vi "Find Sparks with RF Start Signal.vi"(3 "error in (no error)":errorcluster, 4 "Min Spark Length":i32=5000, 5 "Waveform":dbl[](array[numeric])) -> (0 "error out":errorcluster, 2 "Spark Indicies":i32[](array[numeric]))   [LabVIEW 2012]
panel:
  out "Waveform Graph":dbl[](graph)
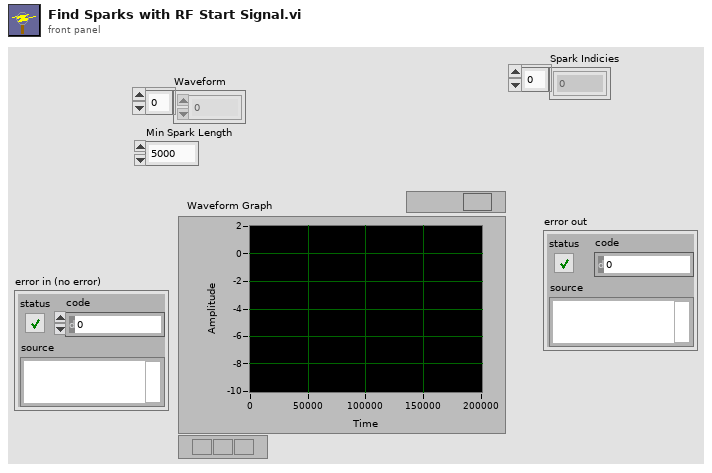
[diagram p1: front panel]
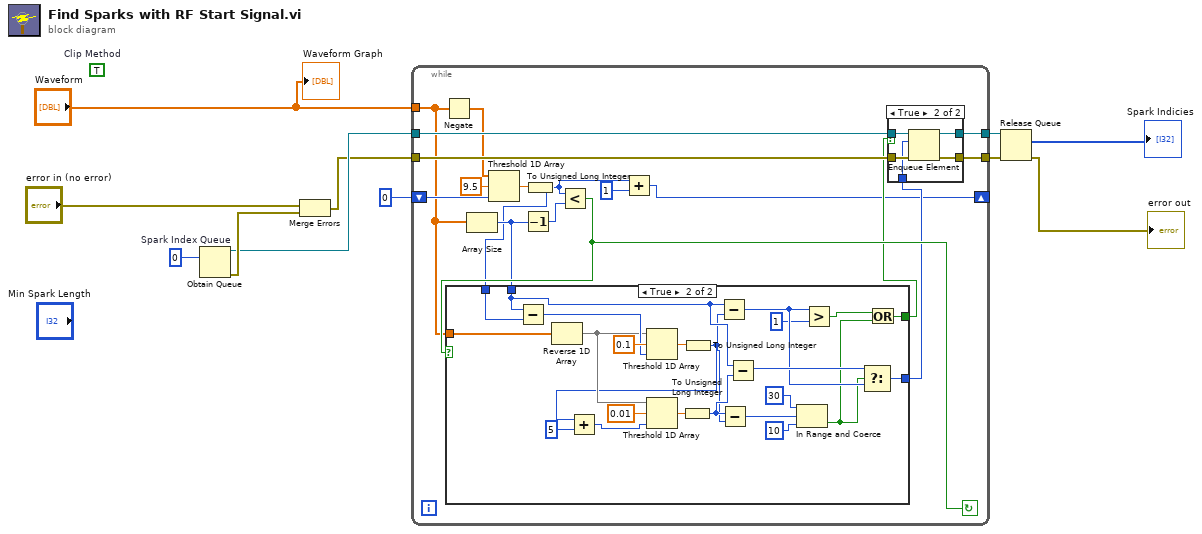
[diagram p0: block diagram]
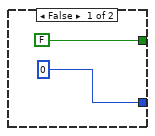
[diagram p3: hidden frame]
diagram:
  (unwired) TRUE  # Clip Method
  n1 = Obtain Queue "Spark Index Queue"(element data type=0 ("# Cluster Levels")) -> (queue out=w6:refnum<queue>, error out=w10:errorcluster)  [unwired: 4 in, 1 out]
  n2 = Merge Errors("error in (no error)", w10) -> (w5:errorcluster)
  n3 = while {
    tunnel: "Waveform" -> [w19]
    shift-right: [w12] -> _
    shift-left: 0 ("start index (0)") -> [w25]
    tunnel: w6 -> [w24]
    tunnel: w5 -> [w23]
    tunnel: [w22] -> w4
    tunnel: [w21] -> w3
    stop <- w20 continue-if-true
    n4 = Negate(x=w19) -> (-x=w15:dbl[])
    n5 = Array Size(array=w19) -> (size(s)=w18:i32)
    n6 = Threshold 1D Array(1:w25, 2:9.5 ("Voltage\nThreshold"), 3:w15) -> (0:w28:dbl)
    n7 = Decrement(x=w18) -> (x-1=w27:i32)
    n8 = To Unsigned Long Integer(number=w28) -> (unsigned 32bit integer=w14:u32)
    n9 = Less?(x=w14, y=w27) -> (x < y?=w20:bool)
    n10 = case shown="True" w20 {
      tunnel: w14 -> [_ w60]
      tunnel: w19 -> [_ w56]
      tunnel: w18 -> [_ w52]
      tunnel: [FALSE w43] -> w17
      tunnel: [u32 0 w46] -> w16
      frame False {
      }
      frame True {
        n11 = Subtract(x=w52, y=w60) -> (x-y=w57:u32)
        n12 = Reverse 1D Array(array=w56) -> (reversed array=w54:dbl[])
        n13 = Threshold 1D Array(1:w57, 2:0.1 ("threshold y"), 3:w54) -> (0:w58:dbl)
        n14 = To Unsigned Long Integer(number=w58) -> (unsigned 32bit integer=w39:u32)
        n15 = Add(x=w39, y=u32 5) -> (x+y=w40:u32)
        n16 = Threshold 1D Array(1:w40, 2:0.01 ("threshold y"), 3:w54) -> (0:w53:dbl)
        n17 = To Unsigned Long Integer(number=w53) -> (unsigned 32bit integer=w51:u32)
        n18 = Subtract(x=w52, y=w39) -> (x-y=w45:u32)
        n19 = Subtract(x=w51, y=w39) -> (x-y=w48:u32)
        n20 = Subtract(x=w52, y=w51) -> (x-y=w47:u32)
        n21 = In Range and Coerce(upper limit=u32 30 ("y"), x=w48, lower limit=u32 10) -> (In Range?=w41:bool)  [unwired: 1 out]
        n22 = Greater?(x=w45, y=u32 1) -> (0:w42:bool)
        n23 = Select(t=w47, s=w41, f=w45) -> (s? t:f=w46:u32)
        n24 = Or(x=w42, y=w41) -> (x .or. y?=w43:bool)
      }
    }
    n25 = Add(x=w14, y=u32 1) -> (x+y=w12:u32)
    n26 = case shown="True" w17 {
      tunnel: w24 -> [w30 w35]
      tunnel: w23 -> [w29 w34]
      tunnel: [w30 w33] -> w22
      tunnel: [w29 w32] -> w21
      tunnel: w16 -> [_ w31]
      frame False {
      }
      frame True {
        n27 = Enqueue Element(queue=w35, element=w31, error in (no error)=w34) -> (queue out=w33:refnum<queue>, error out=w32:errorcluster)  [unwired: 1 in, 1 out]
      }
    }
  }
  n28 = Release Queue(queue=w4, error in (no error)=w3) -> (remaining elements=→"Spark Indicies":i32[], error out=→"error out":errorcluster)  [unwired: 1 in, 1 out]
  "Waveform Graph" <- "Waveform"
